vi "Format Date for SQL.vi"(11 "Date":timestamp) -> (3 "String":string)   [LabVIEW 2018, in "Banking Record.lvclass"]
uses:
  Banking Record.lvclass
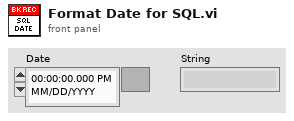
[diagram p1: front panel]
types:
  T1 = typedef "LVDateTimeRec.ctl" = cluster{"fractional second":dbl, "second":i32, "minute":i32, "hour":i32, "day of month":i32, "month":i32, "year":i32, "day of week":i32, "day of year":i32, "DST":i32}
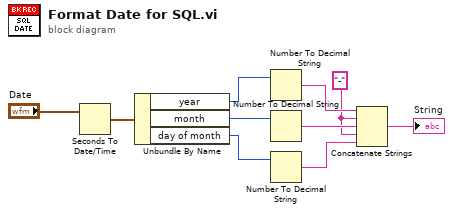
[diagram p0: block diagram]
diagram:
  w7 = "-"
  n1 = Seconds To Date/Time(time stamp (now)="Date") -> (date time rec=w3:T1)  [unwired: 1 in]
  n2 = Unbundle By Name(w3) -> ("year"=w4:i32, "month"=w5:i32, "day of month"=w6:i32)
  n3 = Number To Decimal String(number=w4) -> (decimal integer string=w8:string)  [unwired: 1 in]
  n4 = Number To Decimal String(number=w5) -> (decimal integer string=w9:string)  [unwired: 1 in]
  n5 = Number To Decimal String(number=w6) -> (decimal integer string=w10:string)  [unwired: 1 in]
  n6 = Concatenate Strings(w8, w7, w9, w7, w10) -> (→"String":string)
